vi "LoadModel.vi"(8 "error in (no error)":errorcluster, 10 "Actor In":refnum<class "Actor.lvclass">, 11 "GRMActor in":refnum<class "StepMotorController.lvclass">) -> (0 "error out":errorcluster, 3 "GRMActor out":refnum<class "StepMotorController.lvclass">)   [LabVIEW 2020, in "StepMotorController.lvlib" / "StepMotorController.lvclass"]
uses:
  StepMotorController.lvclass
  <vilib>/ActorFramework/Actor/Actor.lvclass
  Model/Hardware Layer/Simulation Hardware/DemoStepMotor/DemoStepMotor/DemoStepMotor.lvclass
  C:/Program Files/National Instruments/LabVIEW 2020/vi.lib/ActorFramework/Actor/Actor.lvclass
  Model/Hardware Abstraction Layer/Component/GenericActor/GenericActor/GenericController.lvclass
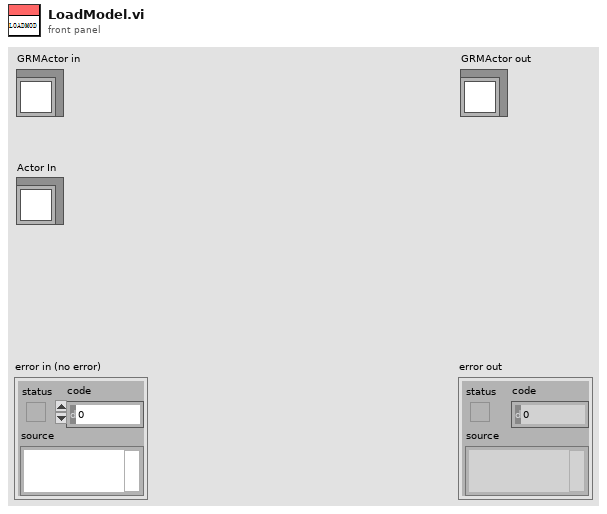
[diagram p1: front panel]
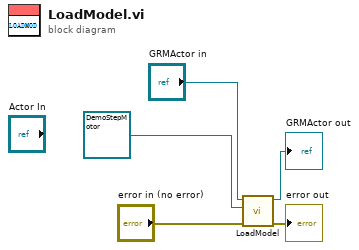
[diagram p0: block diagram]
diagram:
  n1 = call-parent "LoadModel.vi"("error in (no error)"="error in (no error)", "Actor In"=refnum<class "DemoStepMotor.lvclass"> refnum ("DemoStepMotor.lvlib:DemoStepMotor.lvclass"), "GRMActor in"="GRMActor in") -> ("error out"=→"error out":errorcluster, "GRMActor out"=→"GRMActor out":refnum<class "StepMotorController.lvclass">)  [unwired: 7 in]
